vi "1_File_size.vi"() -> ()   [LabVIEW 2014]
uses:
  <vilib>/Utility/file.llb/Write Delimited Spreadsheet (DBL).vi
panel:
  out "Data size":i32 format="%.0f bytes"
  out "TDMS ready":bool
  out "ASCII ready":bool
  out "Bin ready":bool
  out "TDMS delay":u32 format="%.0f ms"
  out "ASCII delay":u32 format="%.0f ms"
  out "binary delay":u32 format="%.0f ms"
  out "TDMS file size":i64 format="%.0f bytes"
  out "ASCII file size":i64 format="%.0f bytes"
  out "binary file size":i64 format="%.0f bytes"
  out "Data":dbl[](array[numeric])
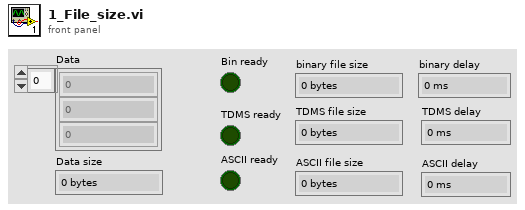
[diagram p1: front panel]
types:
  T1 = enum16{"open", "open or create", "create or replace", "create", "open (read-only)"}
  T2 = enum16{"open", "replace", "create", "open or create", "replace or create", "replace or create with confirmation"}
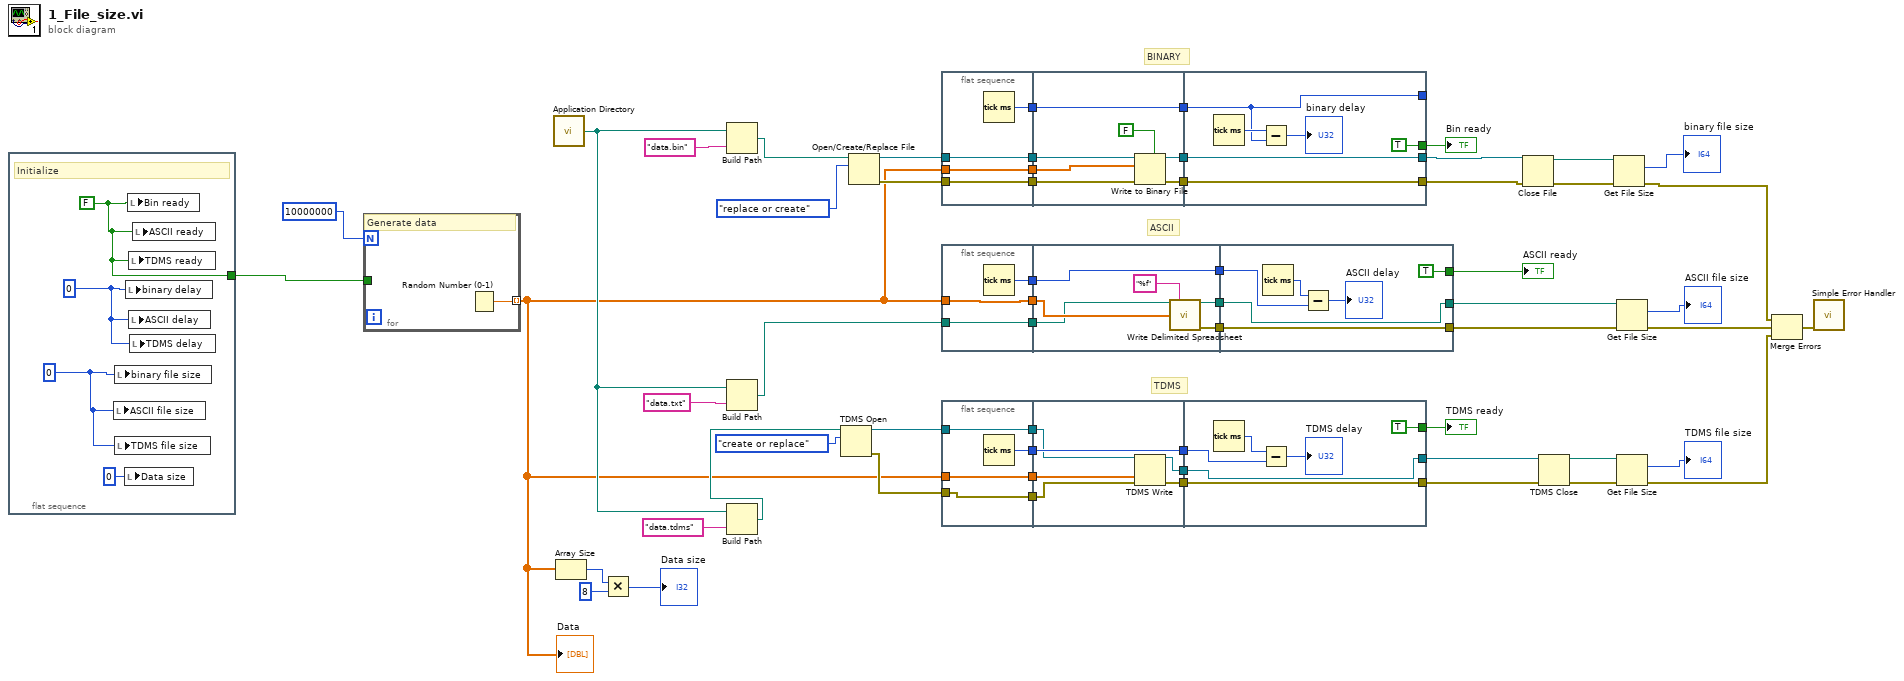
[diagram p0: block diagram]
diagram:
  # "TDMS"
  # "ASCII"
  # "BINARY"
  n1 = flat-sequence {
    tunnel: [w61] -> w5
    frame #0 {
      w62 = i64 0 ("binary file size")
      w63 = u32 0 ("binary delay")
      w61 = FALSE ("Bin ready")
      # "Initialize"
      n2 = local write "ASCII file size"(w62) -> ()
      n3 = local write "binary file size"(w62) -> ()
      n4 = local write "TDMS file size"(w62) -> ()
      n5 = local write "Data size"(0 ("Data size")) -> ()
      n6 = local write "binary delay"(w63) -> ()
      n7 = local write "Bin ready"(w61) -> ()
      n8 = local write "TDMS ready"(w61) -> ()
      n9 = local write "ASCII delay"(w63) -> ()
      n10 = local write "TDMS delay"(w63) -> ()
      n11 = local write "ASCII ready"(w61) -> ()
    }
  }
  n12 = for {
    N: 10000000 -> [_]
    tunnel: [w64] -> w4 mode=indexing
    tunnel: w5 -> [_]
    # "Generate data"
    n13 = Random Number (0-1)() -> (number: 0 to 1=w64:dbl)
  }
  "Data" <- w4
  n14 = call <vilib>:"Application Directory.vi"() -> ("Application Directory"=w49:path)
  n15 = Array Size(array=w4) -> (size(s)=w3:i32)
  n16 = Multiply(x=w3, y=8) -> (x*y=→"Data size":i32)
  n17 = Build Path(base path=w49, name or relative path="data.bin") -> (appended path=w56:path)
  n18 = Build Path(base path=w49, name or relative path="data.txt") -> (appended path=w6:path)
  n19 = Build Path(base path=w49, name or relative path="data.tdms") -> (appended path=w12:path)
  n20 = TDMS Open(10:T1."create or replace" ("operation (0:open)"), 11:w12) -> (0:w9:errorcluster, 3:w11:refnum<k34>)  [unwired: 5 in]
  n21 = Open/Create/Replace File(file path (use dialog)=w56, operation (0:open)=T2."replace or create") -> (refnum out=w54:refnum<file>, error out=w53:errorcluster)  [unwired: 4 in, 1 out]
  n22 = flat-sequence {
    tunnel: w4 -> [w66]
    tunnel: w53 -> [w67]
    tunnel: w54 -> [w68]
    tunnel: [w68] -> w41
    tunnel: [w67] -> w40
    tunnel: [w66] -> w39
    tunnel: [w65] -> w38
    tunnel: w41 -> [w75]
    tunnel: w40 -> [w74]
    tunnel: w39 -> [w73]
    tunnel: w38 -> [w70]
    tunnel: [w72] -> w31
    tunnel: [w71] -> w30
    tunnel: [w70] -> w29
    tunnel: [w78] -> _
    tunnel: [w80] -> w16
    tunnel: [w81] -> w17
    tunnel: w31 -> [w81]
    tunnel: w30 -> [w80]
    tunnel: w29 -> [w78]
    tunnel: [TRUE ("Bin ready")] -> w22
    frame #0 {
      n23 = Tick Count (ms)() -> (millisecond timer value=w65:u32)
    }
    frame #1 {
      n24 = Write to Binary File(file (use dialog)=w75, data=w73, error in=w74, 5:FALSE ("prepend array or string size? (T)")) -> (refnum out=w72:refnum<file>, error out=w71:errorcluster)  [unwired: 2 in, 1 out]
    }
    frame #2 {
      n25 = Tick Count (ms)() -> (millisecond timer value=w79:u32)
      n26 = Subtract(x=w79, y=w78) -> (x-y=→"binary delay":u32)
    }
  }
  n27 = flat-sequence {
    tunnel: [w84] -> w37
    tunnel: w4 -> [w83]
    tunnel: [w83] -> w18
    tunnel: w6 -> [w82]
    tunnel: [w82] -> w7
    tunnel: w37 -> [w90]
    tunnel: [w90] -> w28
    tunnel: [w88] -> w27
    tunnel: [w87] -> w26
    tunnel: w18 -> [w86]
    tunnel: w7 -> [w85]
    tunnel: [w95] -> w35
    tunnel: [w96] -> w36
    tunnel: w28 -> [w92]
    tunnel: w27 -> [w96]
    tunnel: w26 -> [w95]
    tunnel: [TRUE ("Bin ready")] -> w21
    frame #0 {
      n28 = Tick Count (ms)() -> (millisecond timer value=w84:u32)
    }
    frame #1 {
      n29 = call-poly <vilib>:"Write Delimited Spreadsheet.vi"("file path (dialog if empty)"=w85, "format (%.3f)"="%f", "1D data"=w86) -> ("new file path (Not A Path if cancelled)"=w87:path, "error out"=w88:errorcluster)  [unwired: 11 in]
    }
    frame #2 {
      n30 = Tick Count (ms)() -> (millisecond timer value=w94:u32)
      n31 = Subtract(x=w94, y=w92) -> (x-y=→"ASCII delay":u32)
    }
  }
  n32 = flat-sequence {
    tunnel: [w100] -> w34
    tunnel: w4 -> [w99]
    tunnel: [w99] -> w19
    tunnel: w11 -> [w98]
    tunnel: [w98] -> w10
    tunnel: w9 -> [w97]
    tunnel: [w97] -> w8
    tunnel: w34 -> [w106]
    tunnel: [w106] -> w25
    tunnel: [w105] -> w24
    tunnel: [w104] -> w23
    tunnel: w19 -> [w103]
    tunnel: w10 -> [w102]
    tunnel: w8 -> [w101]
    tunnel: [w111] -> w32
    tunnel: [w112] -> w33
    tunnel: w25 -> [w108]
    tunnel: w24 -> [w112]
    tunnel: w23 -> [w111]
    tunnel: [TRUE ("Bin ready")] -> w20
    frame #0 {
      n33 = Tick Count (ms)() -> (millisecond timer value=w100:u32)
    }
    frame #1 {
      n34 = TDMS Write(0:w102, 9:w103, 11:w101) -> (4:w105:refnum<k34>, 15:w104:errorcluster)  [unwired: 3 in, 2 out]
    }
    frame #2 {
      n35 = Tick Count (ms)() -> (millisecond timer value=w109:u32)
      n36 = Subtract(x=w109, y=w108) -> (x-y=→"TDMS delay":u32)
    }
  }
  n37 = Close File(refnum=w17, error in=w16) -> (path=w15:path, error out=w14:errorcluster)
  n38 = TDMS Close(8:w32, 11:w33) -> (0:w45:errorcluster, 3:w43:path)
  n39 = Get File Size(file=w15, error in=w14) -> (size (in bytes)=→"binary file size":i64, 0:w13:errorcluster)  [unwired: 1 out]
  n40 = Get File Size(file=w35, error in=w36) -> (size (in bytes)=→"ASCII file size":i64, 0:w47:errorcluster)  [unwired: 1 out]
  n41 = Get File Size(file=w43, error in=w45) -> (size (in bytes)=→"TDMS file size":i64, 0:w44:errorcluster)  [unwired: 1 out]
  n42 = Merge Errors(w13, w47, w44) -> (w50:errorcluster)
  n43 = call <vilib>:"Simple Error Handler.vi"("error in (no error)"=w50) -> ()  [unwired: 4 in, 5 out]
  "Bin ready" <- w22
  "ASCII ready" <- w21
  "TDMS ready" <- w20
